vi "Get Visible.vi"(7 "Hide if children are hidden? [T]":bool=TRUE, 8 "error in (no error)":errorcluster, 11 "IObject in":refnum<class "IObject.lvclass">) -> (0 "error out":errorcluster, 2 "Visible?":bool, 3 "IObject out":refnum<class "IObject.lvclass">, 4 "Item visible?":bool)   [LabVIEW 2013, in "IObject.lvclass"]
uses:
  IObject.lvclass
  IObject.lvclass/IObject.ctl
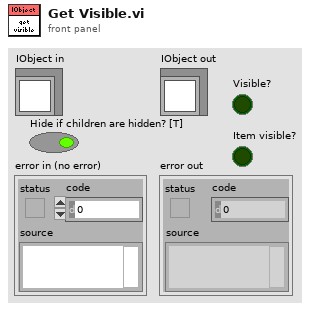
[diagram p1: front panel]
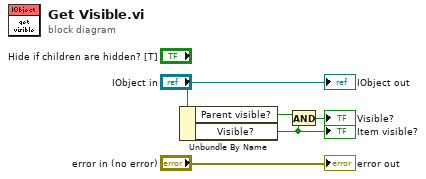
[diagram p0: block diagram]
diagram:
  n1 = Unbundle By Name("IObject in") -> ("Parent visible?"=w2:bool, "Visible?"=w1:bool)
  "Item visible?" <- w1
  n2 = And(x=w2, y=w1) -> (x .and. y?=→"Visible?":bool)
  "error out" <- "error in (no error)"
  "IObject out" <- "IObject in"
